vi "GenericDAQCore.vi"(8 "error in":errorcluster, 9 "SignalBufferQueue":refnum<queue>, 10 "DWFCtrlQueue in":refnum<queue>) -> (0 "error out":errorcluster)   [LabVIEW 2013, in "GenericDAQ.lvlib"]
uses:
  GenericDAQ.lvlib
  <instrlib>/AnalogDiscSDKLv/VIs/DWF_CtrlQueue.ctl
  <instrlib>/AnalogDiscSDKLv/VIs/DWF_State.ctl
  <instrlib>/AnalogDiscSDKLv/VIs/DWF_Signal.ctl
  VI/GenericDAQ_Configs.ctl
  VI/GenericDAQ_PrivateStats.ctl
  VI/GenericDAQ_Status.ctl
  <vilib>/Utility/error.llb/DialogType.ctl
  <instrlib>/GageLv_uic/VI/SetSecondaryDataVIRef_Typedef.ctl
  <vilib>/Utility/error.llb/Error Cluster From Error Code.vi
  <vilib>/ErrorRing/Error Ring.xnode
  <instrlib>/AnalogDiscSDKLv/AnalogDiscSDKLv.lvlib
  <userlib>/Utility/ErrorLog_lib.lvlib
panel:
  in  "StartAll":bool
  out "Core#":i32
  in  "Get_ConfigAll":bool
  out "LiveStat":T1
  in  "GenericDAQ_Config":T3={"Acquisition"={"Sample Rate"=1000000000.0, "Mode"=0, "Start (0)"=0.0, "Depth"=8192.0, "Segment"=1}, "Channels"=[{"Range"=1, "DC Offset"=0}], "Mode(Gage)"=enum."Continuous"} {"Acquisition"."Depth" min=256.0 step=128.0; "Acquisition"."Mode" items=["Single", "Dual", "Quad", "Octal"]; "Acquisition"."Sample Rate" format="%.0p"}
  out "Graph":sgl[][](graph)
  in  "fConfig":bool
  in  "Reset":bool
  in  "CloseAll":bool
  in  "Close":bool
  in  "Enumerate":bool
  in  "Open":bool
  in  "Quit":bool
  in  "Start":bool
  in  "ConfigAll":bool
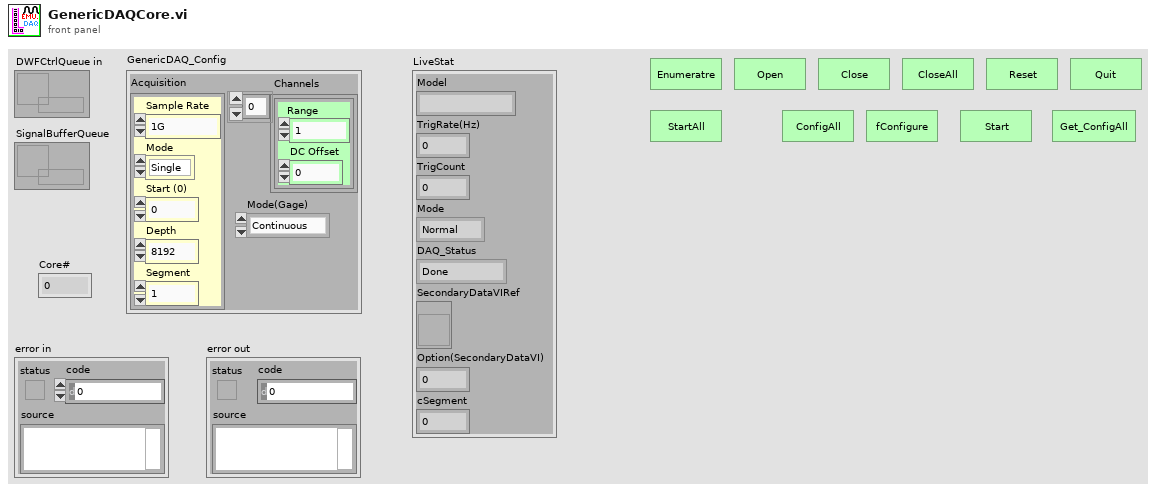
[diagram p1: front panel]
types:
  T1 = typedef "GenericDAQ.lvlib/GenericDAQ_PrivateStats.ctl" = cluster{"Model":string, "TrigRate(Hz)":dbl, "TrigCount":i32, "Mode":enum16{"Normal", "Continuous", "MultiRecord", "HwAverage"}, "DAQ_Status":T2, "SecondaryDataVIRef":refnum<vi>, "Option(SecondaryDataVI)":i32, "cSegment":i32}
  T2 = typedef "GenericDAQ.lvlib/GenericDAQ_Status.ctl" = enum16{"Done", "Armed", "Triggered", "Transfering"}
  T3 = typedef "GenericDAQ.lvlib/GenericDAQ_Configs.ctl" = cluster{"Acquisition":cluster{"Sample Rate":dbl, "Mode":u16, "Start (0)":dbl, "Depth":dbl, "Segment":u32}, "Channels":cluster{"Range":u32, "DC Offset":i32}[], "Mode(Gage)":enum16{"Normal", "Continuous", "MultiRecord", "HwAverage"}}
  T4 = typedef "SetSecondaryDataVIRef_Typedef.ctl" = cluster{"SecondaryDataVIRef.":refnum<vi>, "Option":i32}
  T5 = enum16{"Normal", "MultiRecStart", "MultiRecEnd", "Reserved1", "Reserved2", "Reserved3"}
  T6 = typedef "DialogType.ctl" = u16
  T7 = typedef "AnalogDiscSDKLv.lvlib/DWF_Signal.ctl" = cluster{"tickcount":u32, "Signal":sgl[][], "SecondaryData":dbl[], "Flag":enum16{"Normal", "MultiRecStart", "MultiRecEnd", "Reserved1", "Reserved2", "Reserved3"}}
  T8 = enum16{"Normal", "Continuous", "MultiRecord", "HwAverage"}
  T9 = typedef "AnalogDiscSDKLv.lvlib/DWF_CtrlQueue.ctl" = cluster{"DWF States":T10, "Variant":variant}
  T10 = typedef "AnalogDiscSDKLv.lvlib/DWF_State.ctl" = enum16{"Enumerate", "Open", "Close", "CloseAll", "Reset", "Quit", "==Settings==", "SetAcquisition_", "SetChannels_", "SetTrigger_", "SetAnalogTrigDetector_", "SetAll_AcquChTrig_", "fConfigurate", "fStart", "GetStatus", "_WaitForDone/Idle", "_GetData", "GetAcquisition", "GetChannels", "GetTrigger", "GetAll_AcquChTrig", "==Messaging==", "_PushDataOut", "GetStat_", "GetConfig_", "==ModeSetup==", "SetSignalBuffer_", "SetMode_", "SetSecondaryDataRef._", "==AnalogOut==", "GetChannelCount_AO", "fStart_AO", "SetChEnable_AO", "SetConfig_AO", "SetFuncData_AO", "SetOffset_AO_", "SetMasterNode_AO", "SetStates_AO", "SetSymetry_AO", "SetTriggerSource_AO", "==Trigger==", "ManualTrigger"}
  T11 = cluster{"Handle":u32, "Sample size":u32, "Resolution":i32, "Offset":i32, "Channels":u32, "Boards":u32}
  T12 = cluster{"Sample Rate":dbl, "Mode":u16, "Start (0)":dbl, "Depth":dbl, "Segment":u32}
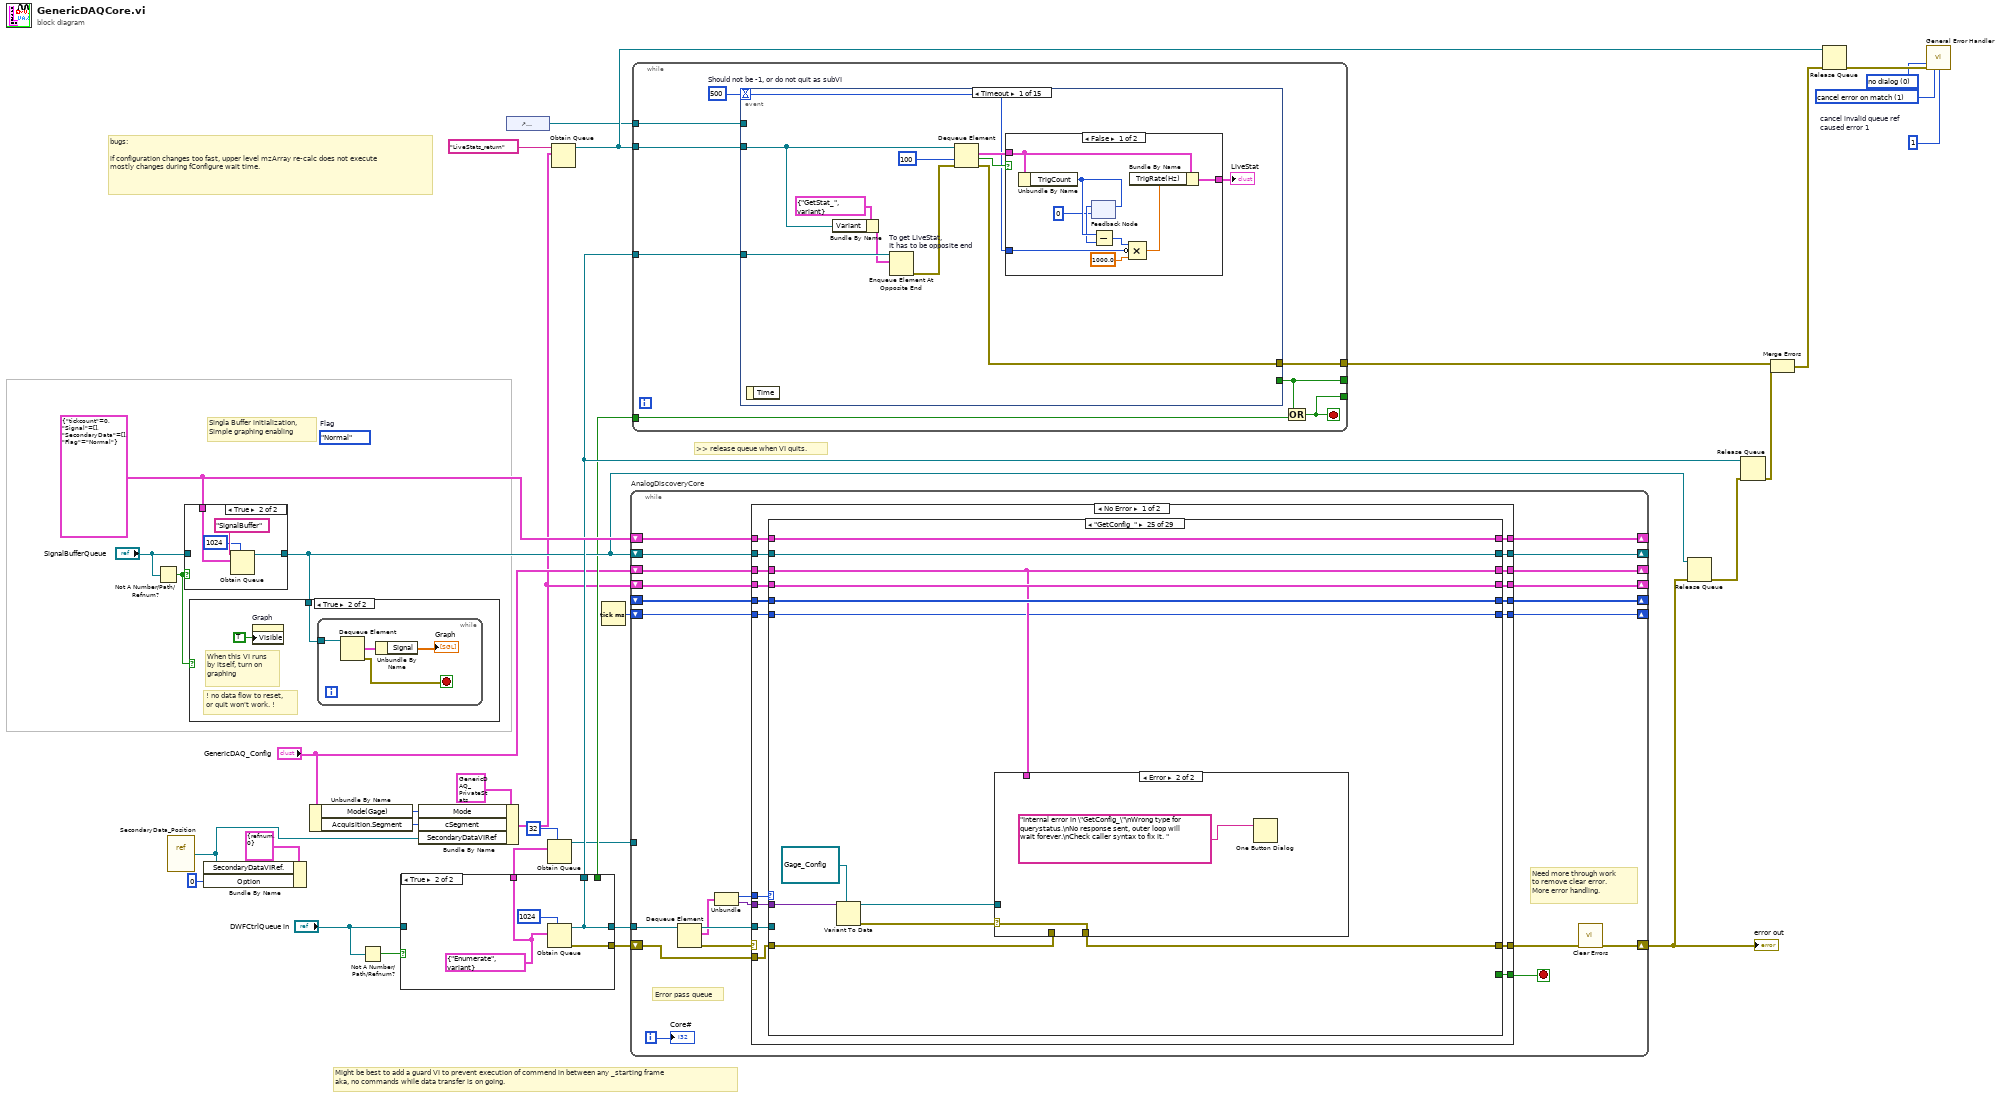
[diagram p0: block diagram]
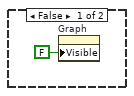
[diagram p2: hidden frame]
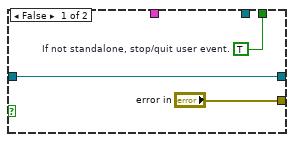
[diagram p4: hidden frame]
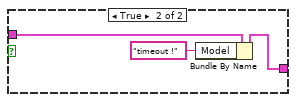
[diagram p5: hidden frame]
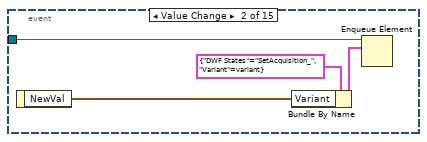
[diagram p6: hidden frame]
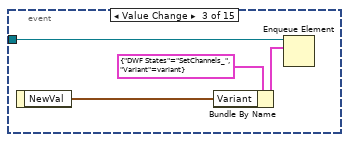
[diagram p7: hidden frame]
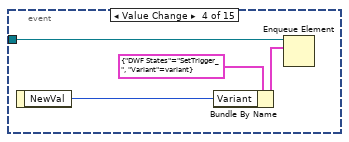
[diagram p8: hidden frame]
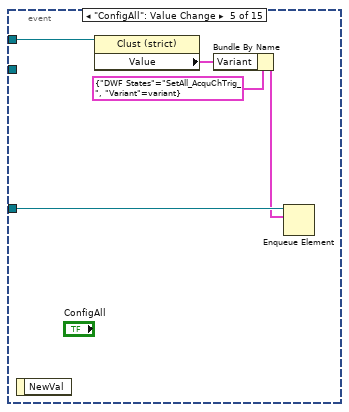
[diagram p9: hidden frame]
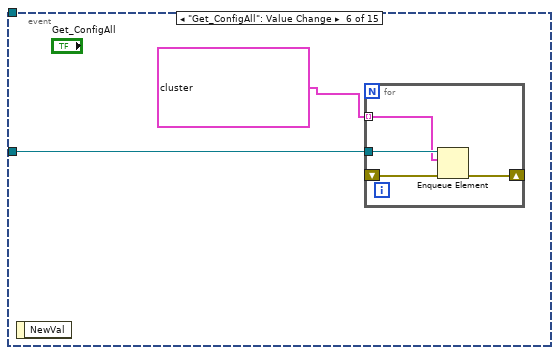
[diagram p10: hidden frame]
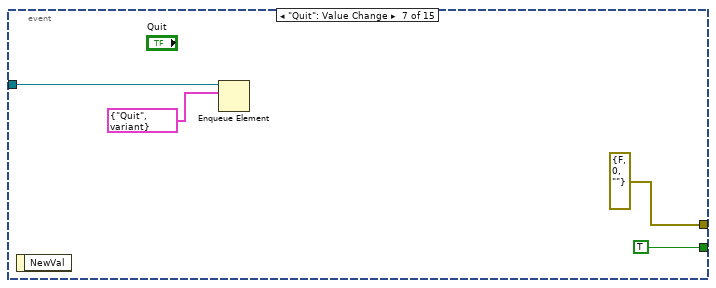
[diagram p11: hidden frame]
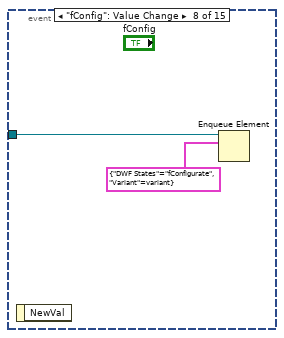
[diagram p12: hidden frame]
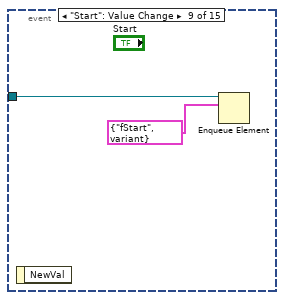
[diagram p13: hidden frame]
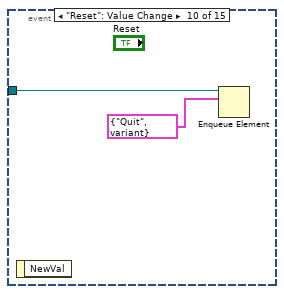
[diagram p14: hidden frame]
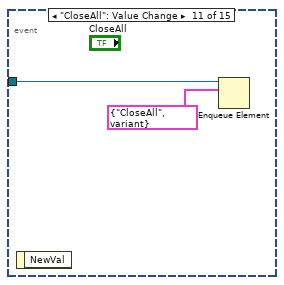
[diagram p15: hidden frame]
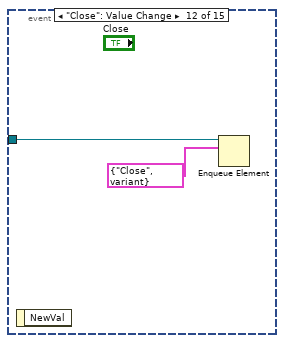
[diagram p16: hidden frame]
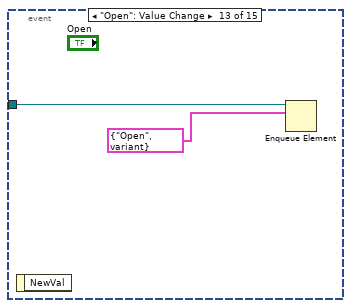
[diagram p17: hidden frame]
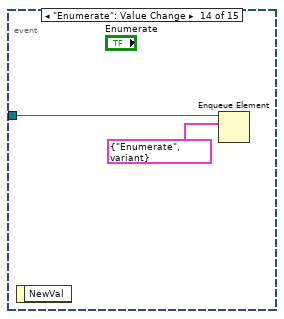
[diagram p18: hidden frame]
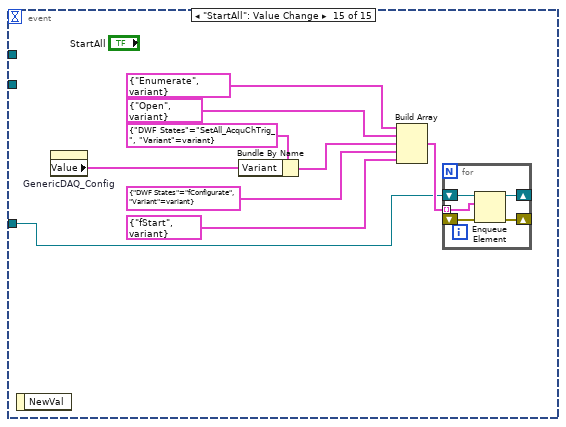
[diagram p19: hidden frame]
diagram:
  (unwired) T5."Normal"  # Flag
  w16 = 1  # cancel invalid queue ref caused error 1
  w17 = 1 items=["no exception", "cancel error on match", "set error on match"] ("[exception action] (none:0)")
  w18 = T6 0 items=["no dialog", "OK message", "continue or stop message", "OK message + warnings", "continue/stop + warnings"] ("type of dialog (OK msg:1)")
  w34 = T7 {"tickcount"=0, "Signal"=[], "SecondaryData"=[], "Flag"=enum."Normal"} ("Signal_Typedef")
  # "Might be best to add a guard VI to prevent execution of commend in between any _starting frame \naka, no commands while data transfer is on going."
  # "bugs:\n\nif configuration changes too fast, upper level mzArray re-calc does not execute\nmostly changes during fConfigure wait time."
  # "Singla Buffer initialization,\nSimple graphing enabling"
  # ">> release queue when VI quits."
  n1 = Not A Number/Path/Refnum?(number/path/refnum="SignalBufferQueue") -> (NaN/Path/Refnum?=w21:bool)
  n2 = vi-ref "SecondaryData_Position.vi"() -> (w1:refnum<vi>)
  n3 = case shown="True" w21 {
    tunnel: w34 -> [_ w39]
    tunnel: [w35 w36] -> w22
    tunnel: "SignalBufferQueue" -> [w35 _]
    frame False {
    }
    frame True {
      n4 = Obtain Queue(max queue size (-1, unlimited)=1024, name (unnamed)="SignalBuffer", element data type=w39) -> (queue out=w36:refnum<queue>)  [unwired: 2 in, 2 out]
    }
  }
  n5 = case shown="True" w21 {
    tunnel: w22 -> [_ w42]
    frame False {
      n6 = property on="Graph" class="WFGraph (strict)"("Visible"=FALSE) -> ()  [unwired: 2 in, 2 out]
    }
    frame True {
      # "! no data flow to reset,\nor quit won't work. !"
      # "When this VI runs\nby itself, turn on \ngraphing"
      n7 = property on="Graph" class="WFGraph (strict)"("Visible"=TRUE) -> ()  [unwired: 2 in, 2 out]
      n8 = while {
        tunnel: w42 -> [w46]
        stop <- w43 stop-if-true
        n9 = Dequeue Element(queue=w46) -> (element=w45:T7, error out=w43:errorcluster)  [unwired: 2 in, 2 out]
        n10 = Unbundle By Name(w45) -> ("Signal"=→"Graph":sgl[][])
      }
    }
  }
  n11 = Bundle By Name(cluster=T4 {"SecondaryDataVIRef."=refnum, "Option"=0} ("SecondaryDataParams."), "SecondaryDataVIRef."=w1, "Option"=0) -> ()  [unwired: 1 out]
  n12 = Unbundle By Name("GenericDAQ_Config") -> ("Mode(Gage)"=w12:T8, "Acquisition.Segment"=w5:u32)
  n13 = Not A Number/Path/Refnum?(number/path/refnum="DWFCtrlQueue in") -> (NaN/Path/Refnum?=w31:bool)
  n14 = case shown="True" w31 {
    tunnel: [w49 w51] -> w33
    tunnel: ["error in" w53] -> w32
    tunnel: "DWFCtrlQueue in" -> [w49 _]
    tunnel: [_ w51] -> w27
    tunnel: [w47 _] -> w15
    tunnel: [_ w50] -> w8
    frame False {
      w47 = TRUE  # If not standalone, stop/quit user event.
    }
    frame True {
      w50 = T9 {"DWF States"=enum."Enumerate", "Variant"=variant}
      n15 = Obtain Queue(max queue size (-1, unlimited)=1024, element data type=w50) -> (queue out=w51:refnum<queue>, error out=w53:errorcluster)  [unwired: 3 in, 1 out]
    }
  }
  n16 = Bundle By Name(cluster=T1 {"Model"="", "TrigRate(Hz)"=0.0, "TrigCount"=0, "Mode"=enum."Normal", "DAQ_Status"=enum."Done", "SecondaryDataVIRef"=refnum, "Option(SecondaryDataVI)"=0, "cSegment"=0} ("PrivateStats(Live)"), "Mode"=w12, "cSegment"=w5, "SecondaryDataVIRef"=w1) -> (w9:T1)
  n17 = control-ref of="GenericDAQ_Config"() -> (w10:refnum<vi>)
  n18 = Obtain Queue(max queue size (-1, unlimited)=32, element data type=w8) -> (queue out=w7:refnum<queue>)  [unwired: 3 in, 2 out]
  n19 = Obtain Queue(name (unnamed)="LiveStats_return", element data type=w9) -> (queue out=w25:refnum<queue>)  [unwired: 3 in, 2 out]
  n20 = Tick Count (ms)() -> (millisecond timer value=w4:u32)
  n21 = while "AnalogDiscoveryCore" {
    shift-right: [w75] -> _
    shift-left: w22 -> [w76]
    tunnel: w33 -> [w62]
    shift-right: [w56] -> w20
    shift-left: w32 -> [w64]
    shift-right: [w73] -> _
    shift-left: "GenericDAQ_Config" -> [w72]
    shift-right: [w60] -> _
    shift-left: w9 -> [w71]
    shift-right: [w65] -> _
    shift-left: _ -> [w69]
    shift-right: [w66] -> _
    shift-left: w34 -> [w70]
    tunnel: w7 -> [_]
    shift-right: [w54] -> _
    shift-left: w4 -> [w55]
    i -> [w58]
    stop <- w74 stop-if-true
    # "Need more through work\nto remove clear error.\nMore error handling."
    # "Error pass queue"
    n22 = Dequeue Element(queue=w62) -> (queue out=w61:refnum<queue>, element=w59:T9, error out=w63:errorcluster)  [unwired: 2 in, 1 out]
    n23 = Unbundle(w59) -> ("DWF States"=w68:T10, "Variant"=w67:variant)
    n24 = case shown="No Error" w63 {
      tunnel: w76 -> [w94 w701]
      tunnel: [w93 w701] -> w75
      tunnel: [w92 TRUE] -> w74
      tunnel: [w91 w699] -> w57
      tunnel: [w90 w702] -> w73
      tunnel: w72 -> [w89 w702]
      tunnel: w71 -> [w88 w703]
      tunnel: w70 -> [w87 w700]
      tunnel: w69 -> [w86 w704]
      tunnel: w61 -> [w85 _]
      tunnel: w68 -> [w84 _]
      tunnel: w67 -> [w83 _]
      tunnel: [w82 w700] -> w66
      tunnel: [w81 w704] -> w65
      tunnel: [w80 w703] -> w60
      tunnel: w64 -> [w79 _]
      tunnel: w55 -> [w78 w698]
      tunnel: [w77 w698] -> w54
      frame No Error {
        n25 = case shown="\"GetConfig_\"" w84 {
          tunnel: w94 -> [w101 w108 w132 w140 w149 w163 w175 w182 w201 w232 w253 w265 w305 w336 w370 w401 w451 w503 w512 w519 w529 w540 w563 w601 w613 w626 w638 w662 w674]
          tunnel: [w101 w108 w132 w140 w149 w163 w175 w182 w201 w232 w253 w265 w305 w336 w370 w401 w451 w503 w512 w519 w529 w540 w563 w601 w613 w626 w639 w662 w674] -> w93
          tunnel: [_ _ _ _ _ _ TRUE _ _ _ _ _ _ _ _ _ _ _ _ _ _ _ _ _ _ _ _ _ _] -> w92
          tunnel: w85 -> [_ _ _ _ _ w159 _ _ _ _ _ w262 w294 w330 _ w403 w447 _ _ _ w524 _ w559 _ _ _ _ _ _]
          tunnel: w79 -> [w100 w104 w128 w134 w148 w158 w170 _ w193 w223 _ w256 w295 w327 w366 w402 w445 w502 w511 w518 w523 _ w561 w595 w604 _ w635 w652 _]
          tunnel: [w100 w104 errorcluster {"status"=FALSE, "code"=0, "source"=""} ("error out") w134 w148 w157 w170 w177 w189 w224 errorcluster {"status"=FALSE, "code"=0, "source"=""} ("error out") w261 w293 w331 w366 w396 w448 w502 w511 w518 w522 w535 w560 w594 w605 w621 w636 w653 w664] -> w91
          tunnel: [w99 w107 w131 w139 w147 w162 w174 w181 w198 w229 w249 w259 w304 w335 w369 w400 w453 w498 w508 w517 w525 w539 w557 w593 w606 w625 w644 w661 w673] -> w90
          tunnel: w89 -> [w99 w107 w131 w139 w147 w162 w174 w181 w196 w227 w249 w259 w304 w335 w369 w400 w453 w497 w506 w517 w525 w539 w557 w593 w606 w625 w644 w661 w673]
          tunnel: [w98 w106 w124 w136 w144 w156 w171 w180 w199 w230 w251 w255 w302 w333 w365 w393 w427 w499 w507 w514 w528 w538 w555 w592 w612 w624 w643 w658 w670] -> w80
          tunnel: w88 -> [w98 w106 w129 w137 w144 w156 w171 w180 w199 w230 w251 w255 w302 w333 w364 w394 w442 w499 w507 w514 w528 w538 w556 w592 w612 w624 w643 w657 w665]
          tunnel: w87 -> [w97 w105 w130 w138 w146 w161 w173 w179 w200 w231 w252 w264 w303 w334 w368 w399 w450 w501 w510 w516 w527 w537 w549 w600 w611 w623 w642 w660 w672]
          tunnel: w86 -> [w96 w103 _ w135 w145 w160 w172 w178 w190 w221 w250 w263 w301 w329 w367 w395 w452 w500 w509 w515 w526 w536 w547 w599 w610 w622 w641 w659 w671]
          tunnel: w83 -> [_ _ w127 _ _ _ _ _ w197 w228 _ w260 _ _ _ _ _ _ _ _ _ _ _ w596 w609 _ w640 w656 w668]
          tunnel: [w97 w105 w130 w138 w146 w161 w173 w179 w200 w231 w252 w264 w303 w334 w368 w399 w449 w501 w510 w516 w527 w537 w549 w600 w611 w623 w642 w660 w672] -> w82
          tunnel: [w96 w103 w115 w135 w145 w160 w172 w178 w191 w221 w250 w263 w301 w329 w367 w395 w444 w500 w509 w515 w526 w536 w547 w599 w610 w622 w641 w659 w671] -> w81
          tunnel: w78 -> [w95 w102 w109 w133 w143 w150 w169 w176 w188 w220 w247 w254 w292 w321 w352 w372 w425 w495 w504 w513 w520 w534 w546 w590 w602 w620 w632 w650 w663]
          tunnel: [w95 w102 w109 w133 w143 w150 w169 w176 w188 w220 w247 w254 w292 w321 w352 w375 w425 w495 w504 w513 w520 w534 w546 w590 w602 w620 w632 w650 w663] -> w77
          frame Default {
          }
          frame "Enumerate" {
          }
          frame "Open" {
            (unwired) T11 {"Handle"=0, "Sample size"=1, "Resolution"=256, "Offset"=0, "Channels"=0, "Boards"=0} ("Handle")
            w113 = 8192 ("dimension size")
            w114 = 2 ("16KSa, per spec")
            n26 = Variant To Data(error in=w128, type="", Variant=w127) -> (data=w123:string, error out=w125:errorcluster)
            n27 = Select(t="any", s=TRUE, f=w123) -> (s? t:f=w110:string)
            n28 = Wait (ms)(milliseconds to wait=u32 0) -> ()  [unwired: 1 out]
            n29 = Bundle By Name(cluster=w125, "source"=w110) -> ()  [unwired: 1 out]
            n30 = Bundle By Name(cluster=w129, "Model"=w110, "TrigRate(Hz)"=0.0, "TrigCount"=0) -> (w124:T1)
            n31 = Initialize Array(0 ("Numeric"), w114, w113) -> (w115:i32[][])
            n32 = Initialize Array(i16 0 ("Numeric"), w114, w113) -> ()  [unwired: 1 out]
            n33 = Initialize Array(u8 0 ("Numeric"), w114, w113) -> ()  [unwired: 1 out]
          }
          frame "Close" {
            n34 = disable-structure shown="Enabled" {
              disable-tunnel: w137 -> [w141 w142]
              disable-tunnel: [w141 w142] -> w136
              frame Enabled {
              }
              frame Disabled {
              }
            }
          }
          frame "CloseAll" {
          }
          frame "Reset" {
            n35 = Unbundle By Name(w156) -> ("Model"=w154:string)
            n36 = Bundle By Name(cluster=T9 {"DWF States"=enum."Open", "Variant"=variant} ("element"), "Variant"=w154) -> (w153:T9)
            n37 = Build Array(w153, T9 {"DWF States"=enum."Close", "Variant"=variant} ("element")) -> (w151:T9[])
            n38 = for {
              tunnel: w159 -> [w167]
              tunnel: w151 -> [w164] mode=indexing
              shift-right: [w165] -> w157
              shift-left: w158 -> [w166]
              n39 = Enqueue Element At Opposite End(queue=w167, element=w164, error in (no error)=w166) -> (error out=w165:errorcluster)  [unwired: 1 in, 2 out]
            }
          }
          frame "Quit" {
          }
          frame "==Settings==" {
            # "Invalid frame"
            n40 = xnode "Error Ring"() -> ("error out"=w177:errorcluster)
          }
          frame "SetAcquisition_" {
            n41 = Unbundle By Name(w196) -> ("Acquisition"=w195:T12)
            n42 = Variant To Data(error in=w193, type=w195, Variant=w197) -> (data=w194:T12, error out=w192:errorcluster)
            n43 = Bundle By Name(cluster=w196, "Acquisition"=w194) -> (w198:T3)
            n44 = case shown="No Error" w192 {
              selector: w192 -> [w203 _]
              tunnel: w199 -> [_ _]
              tunnel: w194 -> [w208 _]
              tunnel: [w205 w214] -> w191
              tunnel: w190 -> [_ w214]
              tunnel: [w203 w213] -> w189
              frame No Error {
                n45 = Unbundle By Name(w208) -> ("Depth"=w207:dbl)
                n46 = flat-sequence {
                  frame #0 {
                    n47 = Wait (ms)(milliseconds to wait=u32 0) -> ()  [unwired: 1 out]
                  }
                }
                n48 = To Long Integer(number=w207) -> (32bit integer=w206:i32)
                n49 = In Range and Coerce(upper limit=512000, x=w206, lower limit=1) -> (coerced(x)=w204:i32)  [unwired: 1 out]
                n50 = Initialize Array(0 ("Numeric"), 1 ("dimension size"), w204) -> (w205:i32[][])
              }
              frame Error {
                n51 = xnode "Error Ring"() -> ("error out"=w213:errorcluster)
              }
            }
          }
          frame "SetChannels_" {
            n52 = Unbundle By Name(w227) -> ("Channels"=w226:cluster{"Range":u32, "DC Offset":i32}[])
            n53 = Variant To Data(error in=w223, type=w226, Variant=w228) -> (data=w225:cluster{"Range":u32, "DC Offset":i32}[], error out=w222:errorcluster)
            n54 = Bundle By Name(cluster=w227, "Channels"=w225) -> (w229:T3)
            n55 = case shown="No Error" w222 {
              selector: w222 -> [w233 _]
              tunnel: w230 -> [_ _]
              tunnel: w225 -> [w235 _]
              tunnel: [w234 w241] -> w224
              frame No Error {
                n56 = for {
                  tunnel: w235 -> [w237] mode=indexing
                  shift-right: [w240] -> w234
                  shift-left: w233 -> [w240]
                  tunnel: [w236] -> _ mode=indexing
                  n57 = Unbundle By Name(w237) -> ("Range"=w238:u32, "DC Offset"=w239:i32)
                  n58 = Bundle("Range"=w238, "DC Offset"=w239) -> (w236:cluster{"Range":u32, "DC Offset":i32})  [unwired: 1 in]
                }
              }
              frame Error {
                n59 = xnode "Error Ring"() -> ("error out"=w241:errorcluster)
              }
            }
          }
          frame "SetTrigger_" {
          }
          frame "SetAll_AcquChTrig_" {
            n60 = Variant To Data(type=w259, Variant=w260) -> (data=w257:T3, error out=w258:errorcluster)  [unwired: 1 in]
            n61 = case shown="No Error" w258 {
              tunnel: w262 -> [w281 _]
              tunnel: [w280 w286] -> w261
              tunnel: w257 -> [w279 _]
              tunnel: w256 -> [w278 _]
              frame No Error {
                n62 = Unbundle By Name(w279) -> ("Mode(Gage)"=w270:T8, "Acquisition"=w276:T12, "Channels"=w274:cluster{"Range":u32, "DC Offset":i32}[])
                n63 = Bundle By Name(cluster=T9 {"DWF States"=enum."SetMode_", "Variant"=variant} ("element"), "Variant"=w270) -> (w267:T9)
                n64 = Bundle By Name(cluster=T9 {"DWF States"=enum."SetAcquisition_", "Variant"=variant} ("element"), "Variant"=w276) -> (w268:T9)
                n65 = Bundle By Name(cluster=T9 {"DWF States"=enum."SetChannels_", "Variant"=variant} ("element"), "Variant"=w274) -> (w266:T9)
                n66 = Build Array(w267, w268, w266, T9 {"DWF States"=enum."SetTrigger_", "Variant"=variant} ("element")) -> (w272:T9[])
                n67 = Reverse 1D Array(array=w272) -> (reversed array=w269:T9[])
                n68 = for "Has to be at the \nopposite end, otherwise\nrace condition" {
                  tunnel: w281 -> [w285]
                  shift-right: [w284] -> w280
                  shift-left: w278 -> [w283]
                  tunnel: w269 -> [w282] mode=indexing
                  n69 = Enqueue Element At Opposite End(queue=w285, element=w282, error in (no error)=w283) -> (error out=w284:errorcluster)  [unwired: 1 in, 2 out]
                }
              }
              frame Error {
                n70 = xnode "Error Ring"() -> ("error out"=w286:errorcluster)
              }
            }
          }
          frame "fConfigurate" {
            # "If dependancy of ErrorLog missing, \njust remove errorlog vi."
            n71 = Flush Queue(queue=w294, error in (no error)=w295) -> (queue out=w300:refnum<queue>, remaining elements=w298:T9[], error out=w299:errorcluster)
            n72 = for "Remove unfinished acquisition process" {
              shift-right: [w312] -> _
              shift-left: w300 -> [w313]
              shift-right: [w310] -> w296
              shift-left: w299 -> [w311]
              tunnel: w298 -> [w306] mode=indexing
              tunnel: T9[] [{"DWF States"=enum."_WaitForDone/Idle", "Variant"=variant}, {"DWF States"=enum."_GetData", "Variant"=variant}, {"DWF States"=enum."_PushDataOut", "Variant"=variant}] ("remaining elements") -> [w309]
              n73 = Search 1D Array(1D array=w309, element=w306) -> (index of element=w308:i32)  [unwired: 1 in]
              n74 = Greater Or Equal To 0?(x=w308) -> (x >= 0?=w307:bool)
              n75 = case shown="False" w307 {
                tunnel: w313 -> [w318 w320]
                tunnel: [w317 w320] -> w312
                tunnel: w311 -> [w316 w319]
                tunnel: [w315 w319] -> w310
                tunnel: w306 -> [w314 _]
                frame False {
                  n76 = Enqueue Element(queue=w318, element=w314, error in (no error)=w316) -> (queue out=w317:refnum<queue>, error out=w315:errorcluster)  [unwired: 1 in, 1 out]
                }
                frame True {
                }
              }
            }
            n77 = call <userlib>:"ErrorLog.vi"("error in (no error)"=w296) -> ("error out"=w293:errorcluster)  [unwired: 10 in]
          }
          frame "fStart" {
            n78 = Flush Queue(queue=w330, error in (no error)=w327) -> (queue out=w328:refnum<queue>, remaining elements=w323:T9[], error out=w325:errorcluster)
            n79 = for "Remove unfinished acquisition process" {
              shift-right: [w343] -> w326
              shift-left: w328 -> [w344]
              shift-right: [w341] -> w324
              shift-left: w325 -> [w342]
              tunnel: w323 -> [w337] mode=indexing
              tunnel: T9[] [{"DWF States"=enum."_WaitForDone/Idle", "Variant"=variant}, {"DWF States"=enum."_GetData", "Variant"=variant}, {"DWF States"=enum."_PushDataOut", "Variant"=variant}] ("remaining elements") -> [w340]
              n80 = Search 1D Array(1D array=w340, element=w337) -> (index of element=w339:i32)  [unwired: 1 in]
              n81 = Greater Or Equal To 0?(x=w339) -> (x >= 0?=w338:bool)
              n82 = case shown="False" w338 {
                tunnel: w344 -> [w349 w351]
                tunnel: [w348 w351] -> w343
                tunnel: w342 -> [w347 w350]
                tunnel: [w346 w350] -> w341
                tunnel: w337 -> [w345 _]
                frame False {
                  n83 = Enqueue Element(queue=w349, element=w345, error in (no error)=w347) -> (queue out=w348:refnum<queue>, error out=w346:errorcluster)  [unwired: 1 in, 1 out]
                }
                frame True {
                }
              }
            }
            n84 = Enqueue Element(queue=w326, element=T9 {"DWF States"=enum."_WaitForDone/Idle", "Variant"=variant}, error in (no error)=w324) -> (error out=w331:errorcluster)  [unwired: 1 in, 2 out]
          }
          frame "GetStatus" {
            n85 = Tick Count (ms)() -> (millisecond timer value=w353:u32)
            n86 = Quotient & Remainder(x=u32 1000, y=u32 500) -> (floor(x/y)=w358:u32)  [unwired: 1 out]
            n87 = Subtract(x=w353, y=w352) -> (x-y=w359:u32)
            n88 = Greater?(x=w359, y=w358) -> (0:w357:bool)
            n89 = And(x=w357, y=TRUE) -> (x .and. y?=w355:bool)
            n90 = Select(t=GenericDAQ_Status."Done" ("DAQ_Status"), s=w355, f=GenericDAQ_Status."Armed" ("DAQ_Status")) -> (s? t:f=w356:T2)
            n91 = Bundle By Name(cluster=w364, "DAQ_Status"=w356) -> (w365:T1)
          }
          frame "_WaitForDone/Idle" {
            w376 = TRUE  # For exteranal OnOff control
            w389 = T10[] [enum."Close", enum."CloseAll", enum."Reset", enum."Quit"] items=["Enumerate", "Open", "Close", "CloseAll", "Reset", "Quit", "==Settings==", "SetAcquisition_", "SetChannels_", "SetTrigger_", "SetAnalogTrigDetector_", "SetAll_AcquChTrig_", "fConfigurate", "fStart", "GetStatus", "_WaitForDone/Idle", "_GetData", "GetAcquisition", "GetChannels", "GetTrigger", "GetAll_AcquChTrig", "==Messaging==", "_PushDataOut", "GetStat_", "GetConfig_", "==ModeSetup==", "SetSignalBuffer_", "SetMode_", "SetSecondaryDataRef._", "==AnalogOut==", "GetChannelCount_AO", "fStart_AO", "SetChEnable_AO", "SetConfig_AO", "SetFuncData_AO", "SetOffset_AO_", "SetMasterNode_AO", "SetStates_AO", "SetSymetry_AO", "SetTriggerSource_AO", "==Trigger==", "ManualTrigger"]
            # "Simulate repetition rate"
            # "0 dne\n1 armed\n2 triggered\n3 transfering"
            n92 = Tick Count (ms)() -> (millisecond timer value=w374:u32)
            n93 = Wait (ms)(milliseconds to wait=u32 1) -> ()  [unwired: 1 out]
            n94 = Quotient & Remainder(x=u32 1000, y=u32 200) -> (floor(x/y)=w378:u32)  [unwired: 1 out]
            n95 = Subtract(x=w374, y=w372) -> (x-y=w379:u32)
            n96 = Greater Or Equal?(x=w379, y=w378) -> (x >= y?=w377:bool)
            n97 = And(x=w377, y=w376) -> (x .and. y?=w373:bool)
            n98 = Preview Queue Element(queue=w403, timeout in ms (-1)=0, error in (no error)=w402) -> (queue out=w398:refnum<queue>, element=w391:T9, timed out?=w390:bool, error out=w397:errorcluster)
            n99 = Unbundle(w391) -> ("DWF States"=w386:T10)  [unwired: 1 out]
            n100 = Select(t=GenericDAQ_Status."Done" ("DAQ_Status"), s=w373, f=GenericDAQ_Status."Armed" ("DAQ_Status")) -> (s? t:f=w371:T2)
            n101 = Select(t=w374, s=w373, f=w372) -> (s? t:f=w375:u32)
            n102 = Search 1D Array(1D array=w389, element=w386) -> (index of element=w388:i32)  [unwired: 1 in]
            n103 = Greater Or Equal To 0?(x=w388) -> (x >= 0?=w387:bool)
            n104 = Bundle By Name(cluster=w394, "DAQ_Status"=w371) -> (w393:T1)
            n105 = Compound Arithmetic op=AND(w387, invert w390) -> (w385:bool)
            n106 = case shown="False" w385 {
              tunnel: w398 -> [w407 _]
              tunnel: w397 -> [w406 w424]
              tunnel: [w405 w424] -> w396
              tunnel: w371 -> [w404 _]
              frame False {
                n107 = case shown="\"Triggered\", Default" w404 {
                  tunnel: w407 -> [w408 w419 w423]
                  tunnel: w406 -> [w411 w418 w422]
                  tunnel: [w410 w417 w421] -> w405
                  frame "Armed" {
                    # "armed ??"
                    # "Typically, this is caused by config change\nduring acquisition. \nPush fConfig and fStart to continure  acuisition."
                    # "armed, not configed??"
                    n108 = for {
                      shift-right: [w414] -> w410
                      shift-left: w411 -> [w415]
                      tunnel: T9[] [{"DWF States"=enum."_WaitForDone/Idle", "Variant"=variant}] -> [w413] mode=indexing
                      tunnel: w408 -> [w412]
                      n109 = Enqueue Element(queue=w412, element=w413, error in (no error)=w415) -> (error out=w414:errorcluster)  [unwired: 1 in, 2 out]
                    }
                  }
                  frame "Done" {
                    # "Done"
                    n110 = Enqueue Element(queue=w419, element=T9 {"DWF States"=enum."_GetData", "Variant"=variant}, error in (no error)=w418) -> (error out=w417:errorcluster)  [unwired: 1 in, 2 out]
                  }
                  frame "Triggered", Default {
                    # "triggered"
                    # "triggered, others"
                    n111 = Enqueue Element(queue=w423, element=T9 {"DWF States"=enum."_WaitForDone/Idle", "Variant"=variant}, error in (no error)=w422) -> (error out=w421:errorcluster)  [unwired: 1 in, 2 out]
                  }
                }
              }
              frame True {
              }
            }
          }
          frame "_GetData" {
            n112 = Unbundle By Name(w453) -> ("Acquisition.Segment"=w431:u32, "Channels"=w440:cluster{"Range":u32, "DC Offset":i32}[], "Acquisition.Depth"=w439:dbl, "Acquisition.Start (0)"=w436:dbl)
            n113 = Unbundle By Name(w442) -> ("TrigCount"=w441:i32, "Option(SecondaryDataVI)"=w435:i32, "SecondaryDataVIRef"=w426:refnum<vi>, "cSegment"=w429:i32)
            n114 = Unbundle By Name(w442) -> ("Mode"=w432:T8)
            n115 = Enqueue Element(queue=w447, element=T9 {"DWF States"=enum."_PushDataOut", "Variant"=variant}, error in (no error)=w445) -> (error out=w437:errorcluster)  [unwired: 1 in, 2 out]
            n116 = Array Size(array=w440) -> (size(s)=w438:i32)
            n117 = Decrement(x=w429) -> (x-1=w430:i32)
            n118 = Subtract(x=w431, y=w430) -> (x-y=w433:u32)
            n119 = for {
              N: w438 -> [_]
              tunnel: w452 -> [w493] mode=indexing
              tunnel: [w492] -> w444 mode=indexing
              tunnel: w439 -> [_]
              tunnel: w436 -> [_]
              shift-right: [w494] -> w434
              shift-left: w437 -> [w494]
              tunnel: w433 -> [_]
              tunnel: w426 -> [w491]
              n120 = call "GenerateFakeSignal.vi"("SecondaryDataVIRef"=w491, "Array"=w493) -> ("simulated signal"=w492:i32[])  [unwired: 9 in]
            }
            n121 = Increment(x=w441) -> (x+1=w443:i32)
            n122 = Bundle By Name(cluster=w442, "TrigCount"=w443, "cSegment"=w430) -> (w428:T1)
            n123 = case shown="\"Continuous\", Default" w432 {
              tunnel: w450 -> [w462 w474 w487]
              tunnel: [w461 w474 w486] -> w449
              tunnel: [w457 w473 w482] -> w448
              tunnel: w426 -> [w460 _ w485]
              tunnel: w435 -> [w459 _ w484]
              tunnel: w434 -> [w457 w472 w482]
              tunnel: w430 -> [_ w468 _]
              tunnel: w431 -> [_ w466 _]
              tunnel: w428 -> [w454 w470 w479]
              tunnel: [w454 w469 w479] -> w427
              frame "Continuous", Default {
                n124 = Not A Number/Path/Refnum?(number/path/refnum=w460) -> (NaN/Path/Refnum?=w455:bool)
                n125 = case shown="False" w455 {
                  tunnel: [w465 _] -> w456
                  tunnel: w460 -> [w464 _]
                  tunnel: w459 -> [w463 _]
                  frame False {
                    n126 = call-by-ref "?"(reference=w464, "Option"=w463) -> ("SecondaryData"=w465:dbl[])  [unwired: 11 in, 2 out]
                  }
                  frame True {
                  }
                }
                n127 = Tick Count (ms)() -> (millisecond timer value=w458:u32)
                n128 = Bundle By Name(cluster=w462, "tickcount"=w458, "SecondaryData"=w456) -> (w461:T7)
              }
              frame "MultiRecord" {
                n129 = Increment(x=w468) -> (x+1=w467:i32)
                n130 = case shown="0" w468 {
                  tunnel: [w477 w478] -> w473
                  tunnel: w472 -> [w477 w478]
                  frame 0 {
                    # "End of MultiRecord Transfer, start next"
                  }
                  frame Default {
                  }
                }
                n131 = Equal?(x=w466, y=w467) -> (x = y?=w471:bool)
                n132 = case shown="True" w471 {
                  tunnel: w467 -> [_ _]
                  tunnel: w470 -> [w475 w476]
                  tunnel: [w475 w476] -> w469
                  frame False {
                  }
                  frame True {
                    # "Get TS array at the first record"
                  }
                }
              }
              frame "Normal" {
                n133 = Not A Number/Path/Refnum?(number/path/refnum=w485) -> (NaN/Path/Refnum?=w480:bool)
                n134 = case shown="False" w480 {
                  tunnel: [w490 _] -> w481
                  tunnel: w485 -> [w489 _]
                  tunnel: w484 -> [w488 _]
                  frame False {
                    n135 = call-by-ref "?"(reference=w489, "Option"=w488) -> ("SecondaryData"=w490:dbl[])  [unwired: 11 in, 2 out]
                  }
                  frame True {
                  }
                }
                n136 = Tick Count (ms)() -> (millisecond timer value=w483:u32)
                n137 = Bundle By Name(cluster=w487, "tickcount"=w483, "SecondaryData"=w481) -> (w486:T7)
              }
            }
          }
          frame "GetAcquisition" {
            n138 = Unbundle By Name(w497) -> ("Acquisition.Sample Rate"=w496:dbl)
            n139 = Bundle By Name(cluster=w497, "Acquisition.Sample Rate"=w496) -> (w498:T3)
          }
          frame "GetChannels" {
            n140 = Unbundle By Name(w506) -> ("Channels"=w505:cluster{"Range":u32, "DC Offset":i32}[])
            n141 = Bundle By Name(cluster=w506, "Channels"=w505) -> (w508:T3)
          }
          frame "GetTrigger" {
          }
          frame "GetAll_AcquChTrig" {
            n142 = for "Has to be at the \nopposite end, otherwise\nrace condition" {
              tunnel: w524 -> [w533]
              shift-right: [w532] -> w522
              shift-left: w523 -> [w531]
              tunnel: T9[] [{"DWF States"=enum."GetAcquisition", "Variant"=variant}, {"DWF States"=enum."GetChannels", "Variant"=variant}, {"DWF States"=enum."GetTrigger", "Variant"=variant}] -> [w530] mode=indexing
              n143 = Enqueue Element At Opposite End(queue=w533, element=w530, error in (no error)=w531) -> (error out=w532:errorcluster)  [unwired: 1 in, 2 out]
            }
          }
          frame "==Messaging==" {
            # "Invalid Frame"
            n144 = xnode "Error Ring"() -> ("error out"=w535:errorcluster)
          }
          frame "_PushDataOut" {
            n145 = Unbundle By Name(w557) -> ("Acquisition.Segment"=w554:u32)  [unwired: 1 out]
            n146 = Unbundle By Name(w556) -> ("Mode"=w562:T8)
            n147 = Unbundle By Name(w556) -> ("cSegment"=w553:i32)
            n148 = case shown="\"Continuous\", Default" w562 {
              tunnel: w561 -> [w565 w572 w589]
              tunnel: [w565 w571 w588] -> w560
              tunnel: w559 -> [_ w570 w587]
              tunnel: w556 -> [w564 w568 w586]
              tunnel: [w564 w567 w585] -> w555
              tunnel: w554 -> [_ w566 w577]
              tunnel: w553 -> [_ _ w576]
              tunnel: [_ _ TRUE] -> w551
              tunnel: [_ _ u32 0 ("unsigned 32bit integer")] -> w548
              frame "Normal" {
              }
              frame "Continuous", Default {
                # "In continuous single trigger  mode, \nre-arming is done in \"_GetData\"\n\nNormal mode => no need to re-arming  daq"
                n149 = Enqueue Element(queue=w570, element=T9 {"DWF States"=enum."_WaitForDone/Idle", "Variant"=variant}, error in (no error)=w572) -> (error out=w571:errorcluster)  [unwired: 1 in, 2 out]
                n150 = Bundle By Name(cluster=w568, "cSegment"=w566) -> (w567:T1)
              }
              frame "MultiRecord" {
                w573 = 1000.0 ("y")
                # "3 functions:\n1. retrival of timestamp\n2. reset cSegment counter\n3. decide continue transfer or wait for next round"
                n151 = Subtract(x=w577, y=w576) -> (x-y=w578:u32)
                n152 = Equal To 0?(x=w576) -> (x = 0?=w583:bool)
                n153 = Decrement "Get Index"(x=w578) -> ()  [unwired: 1 out]
                n154 = Select(t=w577, s=w583, f=w576) -> (s? t:f=w584:u32)
                n155 = Select(t=T9 {"DWF States"=enum."_WaitForDone/Idle", "Variant"=variant} ("element"), s=w583, f=T9 {"DWF States"=enum."_GetData", "Variant"=variant} ("element")) -> (s? t:f=w580:T9)
                n156 = Multiply(x=w573, y=w573) -> (x*y=w575:dbl)
                n157 = Bundle By Name(cluster=w586, "cSegment"=w584) -> (w585:T1)
                n158 = Enqueue Element(queue=w587, element=w580, error in (no error)=w589) -> (error out=w588:errorcluster)  [unwired: 1 in, 2 out]
                n159 = To Unsigned Long Integer(number=w575) -> ()  [unwired: 1 out]
              }
            }
            n160 = Unbundle By Name(w549) -> ("tickcount"=w550:u32)
            n161 = Select(t=w548, s=w551, f=w550) -> (s? t:f=w552:u32)
            n162 = Bundle By Name(cluster=w549, "Signal"=w547, "tickcount"=w552) -> (w558:T7)
            n163 = Enqueue Element "Send/Push Data Out"(queue=w563, element=w558) -> ()  [unwired: 2 in, 3 out]
          }
          frame "GetStat_" {
            n164 = Variant To Data(error in=w595, type=refnum<queue> refnum ("queue out"), Variant=w596) -> (data=w598:refnum<queue>, error out=w597:errorcluster)
            n165 = Enqueue Element "Send Core Stat"(queue=w598, element=w592, error in (no error)=w597) -> (error out=w594:errorcluster)  [unwired: 1 in, 2 out]
          }
          frame "GetConfig_" {
            n166 = Variant To Data(type=refnum<queue> refnum ("queue out"), Variant=w609) -> (data=w608:refnum<queue>, error out=w607:errorcluster)  [unwired: 1 in]
            n167 = case shown="Error" w607 {
              selector: w607 -> [_ w619]
              tunnel: w608 -> [w617 _]
              tunnel: w606 -> [w614 _]
              tunnel: [w616 w619] -> w605
              tunnel: w604 -> [w615 _]
              frame No Error {
                n168 = Enqueue Element(queue=w617, element=w614, error in (no error)=w615) -> (error out=w616:errorcluster)  [unwired: 1 in, 2 out]
              }
              frame Error {
                n169 = One Button Dialog(message="Internal error in \"GetConfig_\"\nWrong type for querystatus.\nNo response sent, outer loop will wait forever.\nCheck caller syntax to fix it. ") -> ()  [unwired: 1 in, 1 out]
              }
            }
          }
          frame "==ModeSetup==" {
            n170 = xnode "Error Ring"() -> ("error out"=w621:errorcluster)
          }
          frame "SetSignalBuffer_" {
            n171 = Variant To Data(type=w638, Variant=w640) -> (data=w637:refnum<queue>, error out=w634:errorcluster)  [unwired: 1 in]
            n172 = Select(t=w638, s=w634, f=w637) -> (s? t:f=w639:refnum<queue>)
            n173 = xnode "Error Ring"() -> ("error out"=w633:errorcluster)
            n174 = Select(t=w633, s=w634, f=w635) -> (s? t:f=w636:errorcluster)
          }
          frame "SetMode_" {
            n175 = Unbundle By Name(w657) -> ("Mode"=w655:T8)
            n176 = Variant To Data(error in=w652, type=w655, Variant=w656) -> (data=w654:T8, error out=w653:errorcluster)
            n177 = Select(t=w655, s=w653, f=w654) -> (s? t:f=w651:T8)
            n178 = Bundle By Name(cluster=w657, "Mode"=w651) -> (w658:T1)
          }
          frame "SetSecondaryDataRef._" {
            n179 = Variant To Data(type=T4 {"SecondaryDataVIRef."=refnum, "Option"=0} ("SecondaryDataParams."), Variant=w668) -> (data=w666:T4, error out=w667:errorcluster)  [unwired: 1 in]
            n180 = case shown="No Error" w667 {
              tunnel: w665 -> [w688 w692]
              tunnel: [w687 w692] -> w670
              tunnel: w666 -> [w683 _]
              tunnel: w665 -> [w680 _]
              tunnel: [w675 w691] -> w664
              frame No Error {
                n181 = Unbundle By Name(w680) -> ("SecondaryDataVIRef"=w678:refnum<vi>)
                n182 = Unbundle By Name(w683) -> ("SecondaryDataVIRef."=w682:refnum<vi>, "Option"=w681:i32)
                n183 = Not A Number/Path/Refnum?(number/path/refnum=w678) -> (NaN/Path/Refnum?=w679:bool)
                n184 = case shown="False" w679 {
                  tunnel: w678 -> [w690 _]
                  tunnel: [w689 _] -> w677
                  frame False {
                    n185 = Close Reference(reference=w690) -> (error out=w689:errorcluster)  [unwired: 1 in]
                  }
                  frame True {
                  }
                }
                n186 = property class="VI Interface Type 0"(reference=w682, error in=w677) -> (reference out=w685:refnum<vi>, error out=w676:errorcluster, "Path"=w686:path)
                n187 = Open VI Reference(type specifier VI Refnum (for type only)=w685, vi path=w686, error in (no error)=w676) -> (vi reference=w684:refnum<vi>, error out=w675:errorcluster)  [unwired: 3 in]
                n188 = Bundle By Name(cluster=w688, "SecondaryDataVIRef"=w684, "Option(SecondaryDataVI)"=w681) -> (w687:T1)
              }
              frame Error {
                n189 = xnode "Error Ring"() -> ("error out"=w691:errorcluster)
              }
            }
          }
        }
      }
      frame Error {
        n190 = xnode "Error Ring"() -> ("error out"=w699:errorcluster)
      }
    }
    n191 = call <vilib>:"Clear Errors.vi"("error in (no error)"=w57) -> ("error out"=w56:errorcluster)  [unwired: 6 in]
    "Core#" <- w58
  }
  "error out" <- w20
  n192 = while {
    tunnel: w27 -> [w718]
    tunnel: w10 -> [w717]
    tunnel: w25 -> [w715]
    tunnel: w15 -> [w714]
    tunnel: [w713] -> w13
    tunnel: [w712] -> _
    tunnel: [w711] -> _
    stop <- w711 stop-if-true
    w716 = 500  # Should not be -1, or do not quit as subVI
    n193 = event shown="[0] Timeout" {
      selector: _ -> [_ _ _ _ _ _ _ _ _ _ _ _ _ _ _]
      dyn-events: _ -> [_ _ _ _ _ _ _ _ _ _ _ _ _ _ _]
      timeout: w716 -> [w720 _ _ _ _ _ _ _ _ _ _ _ _ _ _]
      tunnel: w718 -> [w729 w745 w749 w753 w758 w760 w768 w770 w772 w774 w776 w778 w780 w782 w784]
      tunnel: w717 -> [_ _ _ _ w755 _ _ _ _ _ _ _ _ _ _]
      tunnel: w715 -> [w728 _ _ _ _ _ _ _ _ _ _ _ _ _ _]
      tunnel: [_ _ _ _ _ _ TRUE _ _ _ _ _ _ _ _] -> w712
      tunnel: [w727 _ _ _ _ _ errorcluster {"status"=FALSE, "code"=0, "source"=""} ("error constant") _ _ _ _ _ _ _ _] -> w713
      event Timeout {
        n194 = event-data() -> ()  [unwired: 1 in, 1 out]
        n195 = Bundle By Name(cluster=T9 {"DWF States"=enum."GetStat_", "Variant"=variant} ("element"), "Variant"=w728) -> (w725:T9)
        n196 = Enqueue Element At Opposite End "To get LiveStat,\nIt has to be opposite end"(queue=w729, element=w725) -> (error out=w724:errorcluster)  [unwired: 2 in, 2 out]
        n197 = Dequeue Element(queue=w728, timeout in ms (-1)=100, error in (no error)=w724) -> (element=w723:T1, timed out?=w721:bool, error out=w727:errorcluster)  [unwired: 1 out]
        n198 = case shown="False" w721 {
          tunnel: w723 -> [w738 w741]
          tunnel: [w737 w740] -> w722
          tunnel: w720 -> [w733 _]
          frame False {
            n199 = Unbundle By Name(w738) -> ("TrigCount"=w736:i32)
            n200 = feedback-in #1(w736) -> ()
            n201 = feedback #1(0 ("TrigCount")) -> (w735:i32)
            n202 = Subtract(x=w736, y=w735) -> (x-y=w734:i32)
            n203 = Compound Arithmetic op=MULTIPLY(w734, invert w733, 1000.0 ("value")) -> (w731:dbl)
            n204 = Bundle By Name(cluster=w738, "TrigRate(Hz)"=w731) -> (w737:T1)
          }
          frame True {
            n205 = Bundle By Name(cluster=w741, "Model"="timeout !") -> (w740:T1)
          }
        }
        "LiveStat" <- w722
      }
      event Value Change {
        n206 = event-data() -> ("NewVal"=w742:T12)  [unwired: 1 in]
        n207 = Bundle By Name(cluster=T9 {"DWF States"=enum."SetAcquisition_", "Variant"=variant} ("element"), "Variant"=w742) -> (w743:T9)
        n208 = Enqueue Element(queue=w745, element=w743) -> ()  [unwired: 2 in, 3 out]
      }
      event Value Change {
        n209 = event-data() -> ("NewVal"=w746:cluster{"Range":u32, "DC Offset":i32}[])  [unwired: 1 in]
        n210 = Bundle By Name(cluster=T9 {"DWF States"=enum."SetChannels_", "Variant"=variant} ("element"), "Variant"=w746) -> (w747:T9)
        n211 = Enqueue Element(queue=w749, element=w747) -> ()  [unwired: 2 in, 3 out]
      }
      event Value Change {
        n212 = event-data() -> ("NewVal"=w750:T8)  [unwired: 1 in]
        n213 = Bundle By Name(cluster=T9 {"DWF States"=enum."SetTrigger_", "Variant"=variant} ("element"), "Variant"=w750) -> (w751:T9)
        n214 = Enqueue Element(queue=w753, element=w751) -> ()  [unwired: 2 in, 3 out]
      }
      event "ConfigAll": Value Change {
        n215 = event-data() -> ()  [unwired: 1 in, 1 out]
        n216 = property class="Clust (strict)"(reference=w755) -> ("Value"=w754:T3)  [unwired: 1 in, 2 out]
        n217 = Bundle By Name(cluster=T9 {"DWF States"=enum."SetAll_AcquChTrig_", "Variant"=variant} ("element"), "Variant"=w754) -> (w756:T9)
        n218 = Enqueue Element(queue=w758, element=w756) -> ()  [unwired: 2 in, 3 out]
      }
      event "Get_ConfigAll": Value Change {
        n219 = event-data() -> ()  [unwired: 1 in, 1 out]
        n220 = for {
          tunnel: w760 -> [w764]
          shift-right: [w763] -> _
          shift-left: _ -> [w762]
          tunnel: T9[] [{"DWF States"=enum."GetAcquisition", "Variant"=variant}, {"DWF States"=enum."GetChannels", "Variant"=variant}, {"DWF States"=enum."GetTrigger", "Variant"=variant}] -> [w761] mode=indexing
          n221 = Enqueue Element(queue=w764, element=w761, error in (no error)=w762) -> (error out=w763:errorcluster)  [unwired: 1 in, 2 out]
        }
      }
      event "Quit": Value Change {
        n222 = event-data() -> ()  [unwired: 1 in, 1 out]
        n223 = Enqueue Element(queue=w768, element=T9 {"DWF States"=enum."Quit", "Variant"=variant}) -> ()  [unwired: 2 in, 3 out]
      }
      event "fConfig": Value Change {
        n224 = event-data() -> ()  [unwired: 1 in, 1 out]
        n225 = Enqueue Element(queue=w770, element=T9 {"DWF States"=enum."fConfigurate", "Variant"=variant}) -> ()  [unwired: 2 in, 3 out]
      }
      event "Start": Value Change {
        n226 = event-data() -> ()  [unwired: 1 in, 1 out]
        n227 = Enqueue Element(queue=w772, element=T9 {"DWF States"=enum."fStart", "Variant"=variant}) -> ()  [unwired: 2 in, 3 out]
      }
      event "Reset": Value Change {
        n228 = event-data() -> ()  [unwired: 1 in, 1 out]
        n229 = Enqueue Element(queue=w774, element=T9 {"DWF States"=enum."Quit", "Variant"=variant}) -> ()  [unwired: 2 in, 3 out]
      }
      event "CloseAll": Value Change {
        n230 = event-data() -> ()  [unwired: 1 in, 1 out]
        n231 = Enqueue Element(queue=w776, element=T9 {"DWF States"=enum."CloseAll", "Variant"=variant}) -> ()  [unwired: 2 in, 3 out]
      }
      event "Close": Value Change {
        n232 = event-data() -> ()  [unwired: 1 in, 1 out]
        n233 = Enqueue Element(queue=w778, element=T9 {"DWF States"=enum."Close", "Variant"=variant}) -> ()  [unwired: 2 in, 3 out]
      }
      event "Open": Value Change {
        n234 = event-data() -> ()  [unwired: 1 in, 1 out]
        n235 = Enqueue Element(queue=w780, element=T9 {"DWF States"=enum."Open", "Variant"=variant}) -> ()  [unwired: 2 in, 3 out]
      }
      event "Enumerate": Value Change {
        n236 = event-data() -> ()  [unwired: 1 in, 1 out]
        n237 = Enqueue Element(queue=w782, element=T9 {"DWF States"=enum."Enumerate", "Variant"=variant}) -> ()  [unwired: 2 in, 3 out]
      }
      event "StartAll": Value Change {
        n238 = event-data() -> ()  [unwired: 1 in, 1 out]
        n239 = property on="GenericDAQ_Config" class="Clust (strict)"() -> ("Value"=w783:T3)  [unwired: 2 in, 2 out]
        n240 = Bundle By Name(cluster=T9 {"DWF States"=enum."SetAll_AcquChTrig_", "Variant"=variant} ("element"), "Variant"=w783) -> (w788:T9)
        n241 = Build Array(T9 {"DWF States"=enum."Enumerate", "Variant"=variant} ("element"), T9 {"DWF States"=enum."Open", "Variant"=variant} ("element"), w788, T9 {"DWF States"=enum."fConfigurate", "Variant"=variant} ("element"), T9 {"DWF States"=enum."fStart", "Variant"=variant} ("element")) -> (w791:T9[])
        n242 = for {
          shift-right: [w795] -> _
          shift-left: w784 -> [w796]
          tunnel: w791 -> [w794] mode=indexing
          shift-right: [w793] -> _
          shift-left: _ -> [w792]
          n243 = Enqueue Element(queue=w796, element=w794, error in (no error)=w792) -> (queue out=w795:refnum<queue>, error out=w793:errorcluster)  [unwired: 1 in, 1 out]
        }
      }
    }
    n244 = Or(x=w712, y=w714) -> (x .or. y?=w711:bool)
  }
  n245 = Release Queue(queue=w22, error in (no error)=w20) -> (error out=w26:errorcluster)  [unwired: 1 in, 2 out]
  n246 = Release Queue(queue=w27, error in (no error)=w26) -> (error out=w24:errorcluster)  [unwired: 1 in, 2 out]
  n247 = Merge Errors(w13, w24) -> (w14:errorcluster)
  n248 = Release Queue(queue=w25, error in (no error)=w14) -> (error out=w19:errorcluster)  [unwired: 1 in, 2 out]
  n249 = call <vilib>:"General Error Handler.vi"("type of dialog (OK msg:1)"=w18, "error in (no error)"=w19, "[exception action] (none:0)"=w17, "[exception code]"=w16) -> ()  [unwired: 7 in, 5 out]
